vi "getChellChans.vi"(2 "LSB":dbl[](array[numeric]), 3 "MSB":dbl[](array[numeric])) -> (0 "Sample Index":i32[](array[numeric]), 1 "No. Chell Chans.":dbl[](array[numeric]))   [LabVIEW 2013]
uses:
  <vilib>/Analysis/baseanly.llb/Normalize Vector.vi
  Globals/measurementGlobal.vi
  <vilib>/Analysis/NI_AALPro.lvlib
  <vilib>/Analysis/NI_AALBase.lvlib
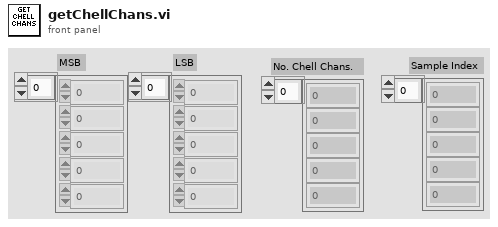
[diagram p1: front panel]
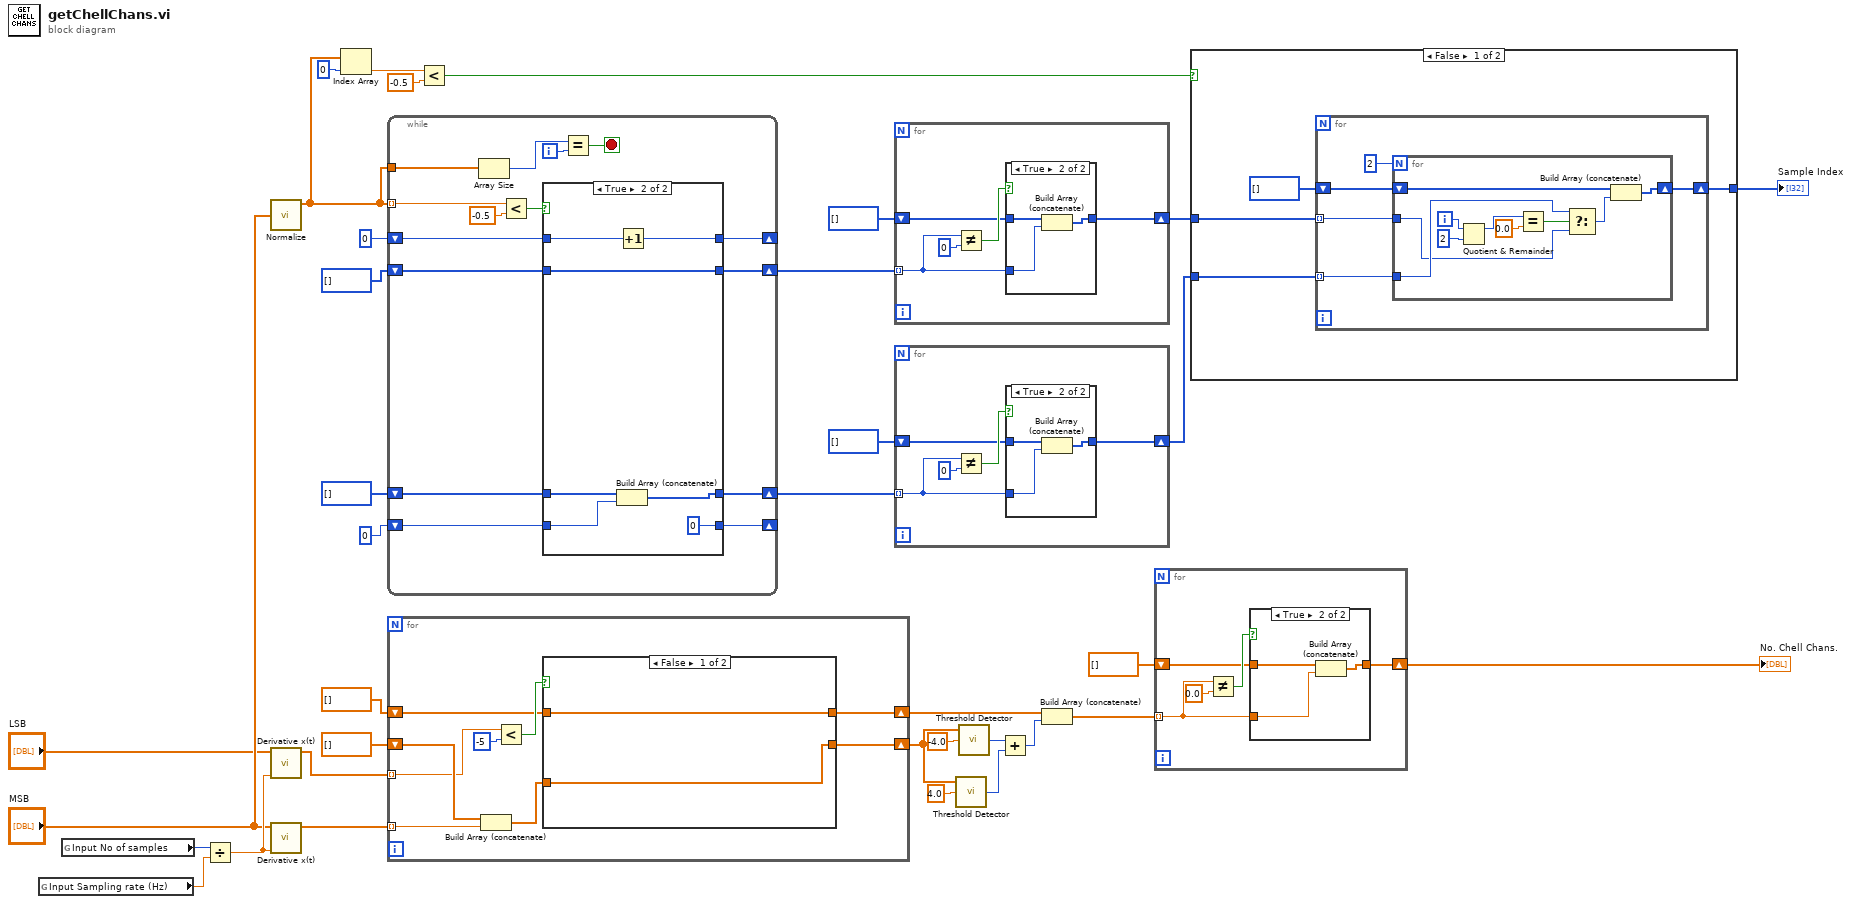
[diagram p0: block diagram]
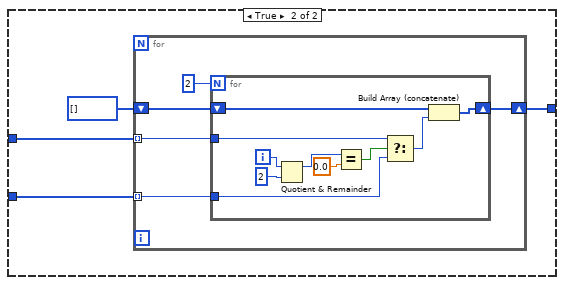
[diagram p2: hidden frame]
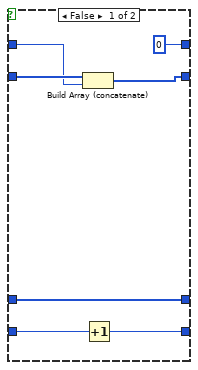
[diagram p5: hidden frame]
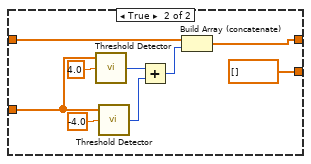
[diagram p7: hidden frame]
diagram:
  n1 = global read "measurementGlobal.vi" "Input Sampling rate (Hz)"() -> (w24:dbl)
  n2 = global read "measurementGlobal.vi" "Input No of samples"() -> (w21:i32)
  n3 = Divide(x=w21, y=w24) -> (x/y=w23:dbl)
  n4 = call-poly <vilib>:"Normalize.vi"("Vector"="MSB") -> ("Normalized Vector"=w9:dbl[])  [unwired: 1 in, 3 out]
  n5 = call <vilib>:"Derivative x(t).vi"("dt"=w23, "X"="LSB") -> ("dX/dt"=w3:dbl[])  [unwired: 8 in, 1 out]
  n6 = call <vilib>:"Derivative x(t).vi"("dt"=w23, "X"="MSB") -> ("dX/dt"=w20:dbl[])  [unwired: 8 in, 1 out]
  n7 = Index Array(array=w9, index=0) -> (element=w7:dbl)
  n8 = while {
    tunnel: w9 -> [w48] mode=indexing
    shift-right: [w46] -> _
    shift-left: 0 -> [w47]
    shift-right: [w44] -> _
    shift-left: 0 -> [w45]
    shift-right: [w38] -> w16
    shift-left: i32[] [] -> [w39]
    tunnel: w9 -> [w42]
    shift-right: [w36] -> w12
    shift-left: i32[] [] -> [w37]
    i -> [w43]
    stop <- w40 stop-if-true
    n9 = Array Size(array=w42) -> (size(s)=w41:i32)
    n10 = Less?(x=w48, y=-0.5) -> (x < y?=w49:bool)
    n11 = case shown="True" w49 {
      tunnel: w47 -> [w53 w64]
      tunnel: [0 w62] -> w46
      tunnel: w45 -> [w57 w59]
      tunnel: [w56 0] -> w44
      tunnel: w39 -> [w55 w61]
      tunnel: [w54 w61] -> w38
      tunnel: w37 -> [w51 w60]
      tunnel: [w51 w58] -> w36
      frame False {
        n12 = Build Array (concatenate)(w55, w53) -> (w54:i32[])
        n13 = Increment(x=w57) -> (x+1=w56:i32)
      }
      frame True {
        n14 = Build Array (concatenate)(w60, w59) -> (w58:i32[])
        n15 = Increment(x=w64) -> (x+1=w62:i32)
      }
    }
    n16 = Equal?(x=w41, y=w43) -> (x = y?=w40:bool)
  }
  n17 = for {
    tunnel: w3 -> [w71] mode=indexing
    tunnel: w20 -> [w73] mode=indexing
    shift-right: [w68] -> w31
    shift-left: dbl[] [] -> [w72]
    shift-right: [w65] -> w22
    shift-left: dbl[] [] -> [w67]
    n18 = Build Array (concatenate)(w72, w73) -> (w66:dbl[])
    n19 = Less?(x=w71, y=-5) -> (x < y?=w69:bool)
    n20 = case shown="False" w69 {
      tunnel: w66 -> [w75 w83]
      tunnel: [w75 dbl[] []] -> w68
      tunnel: w67 -> [w74 w82]
      tunnel: [w74 w81] -> w65
      frame False {
      }
      frame True {
        n21 = call <vilib>:"Threshold Detector.vi"("threshold"=4.0, "X"=w83) -> ("count"=w78:i32)  [unwired: 1 in, 2 out]
        n22 = call <vilib>:"Threshold Detector.vi"("threshold"=-4.0, "X"=w83) -> ("count"=w79:i32)  [unwired: 1 in, 2 out]
        n23 = Add(x=w78, y=w79) -> (x+y=w77:i32)
        n24 = Build Array (concatenate)(w82, w77) -> (w81:dbl[])
      }
    }
  }
  n25 = Less?(x=w7, y=-0.5) -> (x < y?=w10:bool)
  n26 = for {
    tunnel: w16 -> [w86] mode=indexing
    shift-right: [w85] -> w5
    shift-left: i32[] [] -> [w87]
    n27 = Not Equal?(x=w86, y=0) -> (x != y?=w88:bool)
    n28 = case shown="True" w88 {
      tunnel: w87 -> [w90 w93]
      tunnel: w86 -> [_ w92]
      tunnel: [w90 w91] -> w85
      frame False {
      }
      frame True {
        n29 = Build Array (concatenate)(w93, w92) -> (w91:i32[])
      }
    }
  }
  n30 = for {
    tunnel: w12 -> [w95] mode=indexing
    shift-right: [w94] -> w6
    shift-left: i32[] [] -> [w96]
    n31 = Not Equal?(x=w95, y=0) -> (x != y?=w97:bool)
    n32 = case shown="True" w97 {
      tunnel: w96 -> [w99 w102]
      tunnel: w95 -> [_ w101]
      tunnel: [w99 w100] -> w94
      frame False {
      }
      frame True {
        n33 = Build Array (concatenate)(w102, w101) -> (w100:i32[])
      }
    }
  }
  n34 = call <vilib>:"Threshold Detector.vi"("threshold"=4.0, "X"=w31) -> ("count"=w29:i32)  [unwired: 1 in, 2 out]
  n35 = call <vilib>:"Threshold Detector.vi"("threshold"=-4.0, "X"=w31) -> ("count"=w30:i32)  [unwired: 1 in, 2 out]
  n36 = Add(x=w30, y=w29) -> (x+y=w28:i32)
  n37 = Build Array (concatenate)(w22, w28) -> (w27:dbl[])
  n38 = for {
    tunnel: w27 -> [w105] mode=indexing
    shift-right: [w103] -> w25
    shift-left: dbl[] [] -> [w104]
    n39 = Not Equal?(x=w105, y=0.0) -> (x != y?=w106:bool)
    n40 = case shown="True" w106 {
      tunnel: w105 -> [_ w110]
      tunnel: w104 -> [w108 w109]
      tunnel: [w108 w111] -> w103
      frame False {
      }
      frame True {
        n41 = Build Array (concatenate)(w109, w110) -> (w111:dbl[])
      }
    }
  }
  "No. Chell Chans." <- w25
  n42 = case shown="False" w10 {
    tunnel: w6 -> [w115 w133]
    tunnel: w5 -> [w114 w132]
    tunnel: [w112 w131] -> w4
    frame False {
      n43 = for {
        tunnel: w115 -> [w120] mode=indexing
        tunnel: w114 -> [w119] mode=indexing
        shift-right: [w116] -> w112
        shift-left: i32[] [] -> [w117]
        n44 = for {
          N: 2 -> [_]
          tunnel: w119 -> [w121]
          tunnel: w120 -> [w122]
          shift-right: [w126] -> w116
          shift-left: w117 -> [w128]
          i -> [w130]
          n45 = Quotient & Remainder(x=w130, y=2) -> (x-y*floor(x/y)=w124:i32)  [unwired: 1 out]
          n46 = Equal?(x=w124, y=0.0) -> (x = y?=w123:bool)
          n47 = Select(t=w122, s=w123, f=w121) -> (s? t:f=w127:i32)
          n48 = Build Array (concatenate)(w128, w127) -> (w126:i32[])
        }
      }
    }
    frame True {
      n49 = for {
        tunnel: w133 -> [w138] mode=indexing
        tunnel: w132 -> [w137] mode=indexing
        shift-right: [w136] -> w131
        shift-left: i32[] [] -> [w139]
        n50 = for {
          N: 2 -> [_]
          tunnel: w137 -> [w140]
          tunnel: w138 -> [w147]
          shift-right: [w144] -> w136
          shift-left: w139 -> [w146]
          i -> [w149]
          n51 = Quotient & Remainder(x=w149, y=2) -> (x-y*floor(x/y)=w142:i32)  [unwired: 1 out]
          n52 = Equal?(x=w142, y=0.0) -> (x = y?=w141:bool)
          n53 = Select(t=w140, s=w141, f=w147) -> (s? t:f=w145:i32)
          n54 = Build Array (concatenate)(w146, w145) -> (w144:i32[])
        }
      }
    }
  }
  "Sample Index" <- w4
